vi "CNR cauchy model function.vi"(9 "residual ( f(x) )":dbl[](array[numeric]), 10 "h":dbl[](array[numeric]), 11 "Jacobian":T1) -> (1 "L(0)-L(h_dl)":dbl, 3 "L(h_dl)":dbl)   [LabVIEW 2020, in "NI_Gmath.lvlib"]
uses:
  NI_Gmath.lvlib
  RealMatrix.ctl
  NI_AALBase.lvlib
  NI_Matrix.lvlib
panel:
  out "x^2":dbl
  out "L(0)":dbl
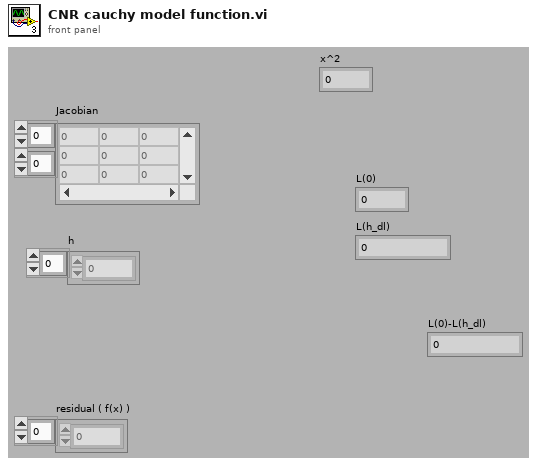
[diagram p1: front panel]
types:
  T1 = typedef "NI_Matrix.lvlib/RealMatrix.ctl" = dbl[][]
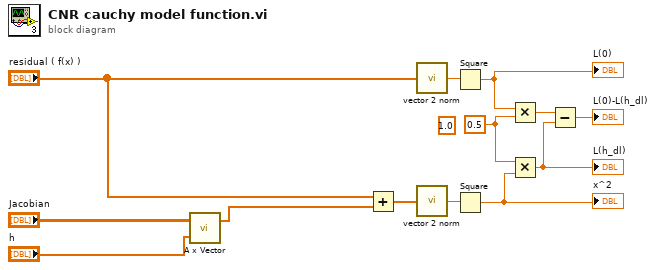
[diagram p0: block diagram]
diagram:
  (unwired) 1.0 ("y")
  w2 = 0.5 ("y")
  n1 = call "A x Vector.vi"("Vector"="h", "A"="Jacobian") -> ("A x Vector"=w1:dbl[])  [unwired: 1 out]
  n2 = Add(x="residual ( f(x) )", y=w1) -> (x+y=w8:dbl[])
  n3 = call "vector 2 norm.vi"("vector"="residual ( f(x) )") -> ("vector2_norm"=w5:dbl)  [unwired: 14 in]
  n4 = call "vector 2 norm.vi"("vector"=w8) -> ("vector2_norm"=w7:dbl)  [unwired: 14 in]
  n5 = Square(x=w5) -> (x^2=w3:dbl)
  "L(0)" <- w3
  n6 = Square(x=w7) -> (x^2=w4:dbl)
  "x^2" <- w4
  n7 = Multiply(x=w3, y=w2) -> (x*y=w10:dbl)
  n8 = Multiply(x=w2, y=w4) -> (x*y=w11:dbl)
  "L(h_dl)" <- w11
  n9 = Subtract(x=w10, y=w11) -> (x-y=→"L(0)-L(h_dl)":dbl)
